vi "SaveStep.vi"(11 "Cluster":T2) -> (1 "StepForward":T1(ring), 2 "StepBack":T1(ring), 3 "Cluster":T2)   [LabVIEW 2021, in "Tree.lvlib" / "Tree.lvclass"]
uses:
  Tree.lvclass
  TreeController.ctl
  TreeData.ctl
panel:
  out "Del index":i32
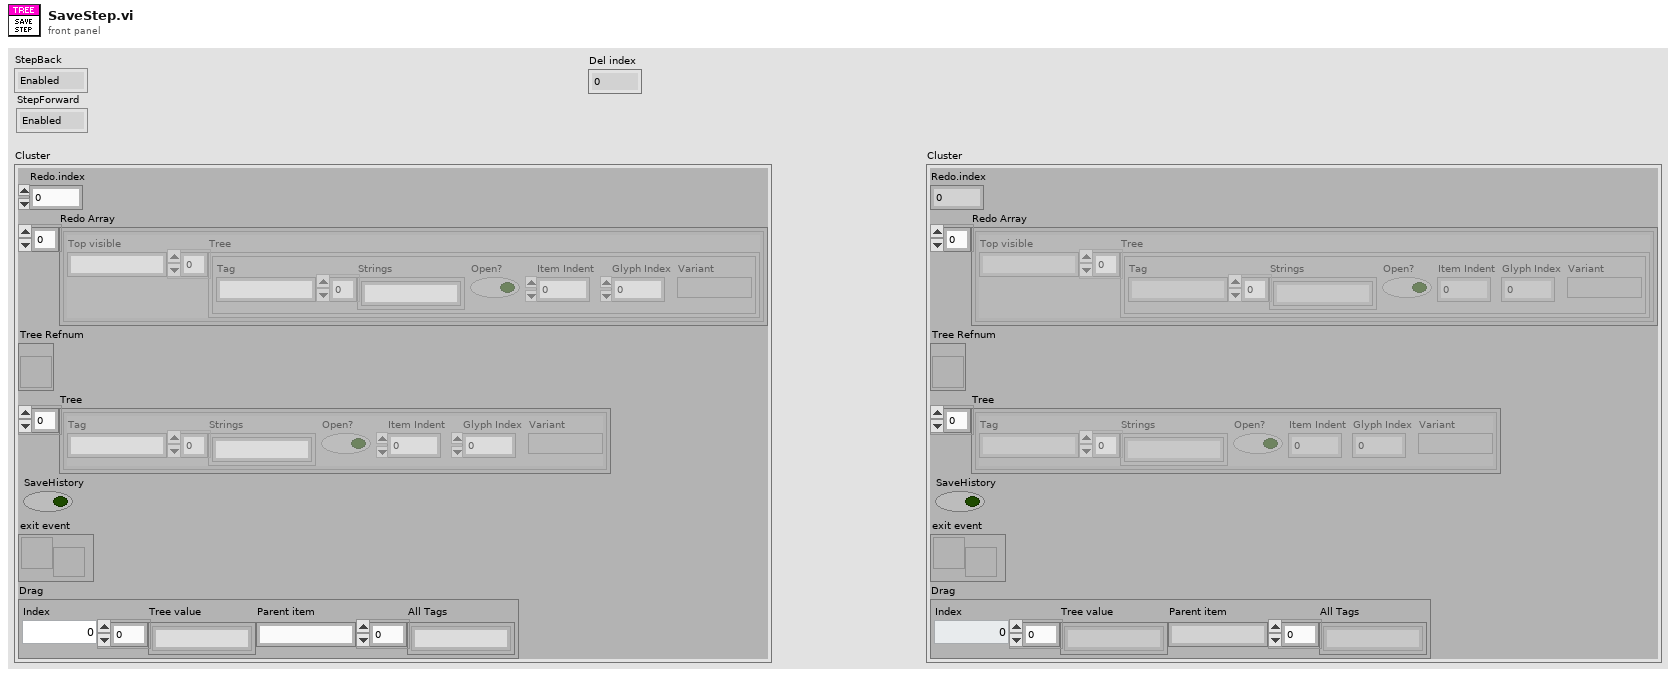
[diagram p1: front panel]
types:
  T1 = enum8{"Enabled", "Disabled", "Disabled and Grayed Out"}
  T2 = typedef "Tree.lvlib/Tree.lvclass/TreeController.ctl" = cluster{"Redo.index":i32, "Redo Array":cluster{"Top visible":string, "Tree":T3[]}[], "Tree Refnum":refnum<vi>, "Tree":T3[], "SaveHistory":bool, "exit event":refnum<user-event>, "Drag":cluster{"Index":i32, "Tree value":string[], "Parent item":string, "All Tags":string[]}}
  T3 = typedef "Tree.lvlib/Tree.lvclass/TreeData.ctl" = cluster{"Tag":string, "Strings":string[], "Open?":bool, "Item Indent":i32, "Glyph Index":i32, "Variant":variant}
  T4 = typedef "LVNodeAndColumnTypeDef.ctl" = cluster{"Node":string, "Column":i32}
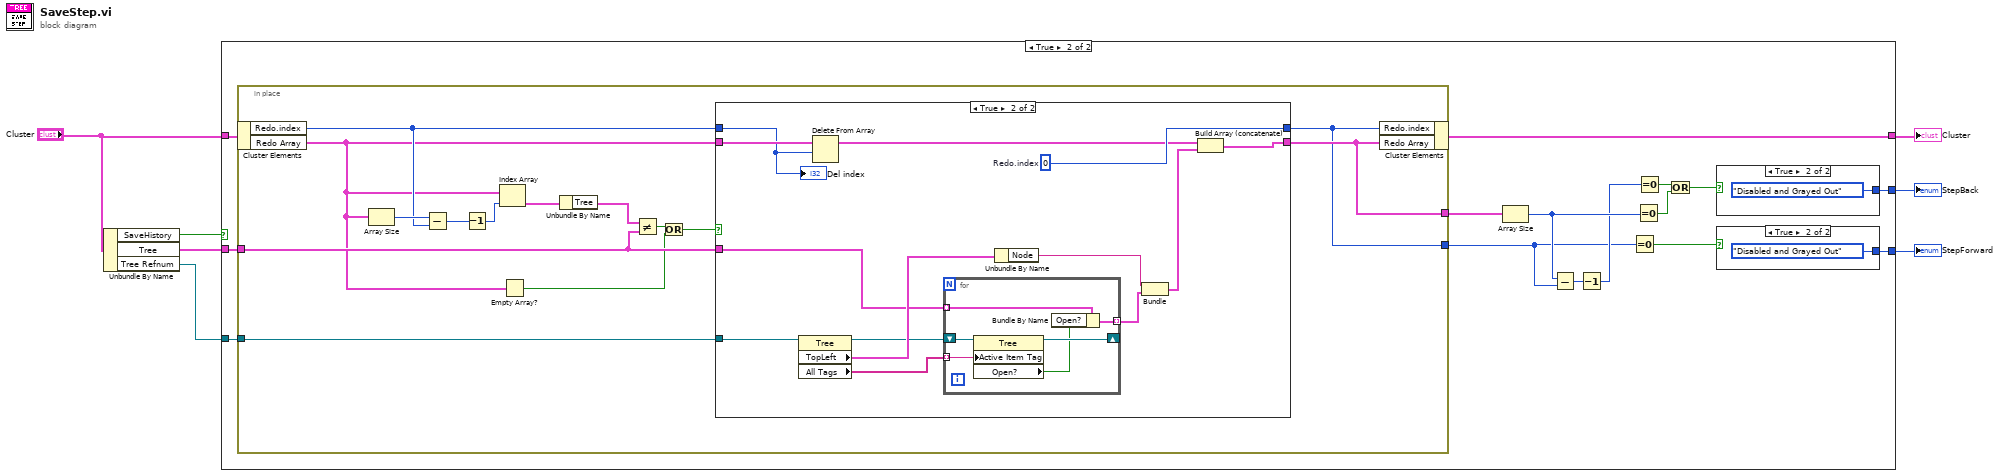
[diagram p0: block diagram]
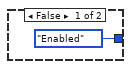
[diagram p3: hidden frame]
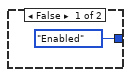
[diagram p4: hidden frame]
diagram:
  n1 = Unbundle By Name("Cluster") -> ("SaveHistory"=w2:bool, "Tree"=w7:T3[], "Tree Refnum"=w1:refnum<vi>)
  n2 = case shown="True" w2 {
    tunnel: w7 -> [_ w23]
    tunnel: "Cluster" -> [w8 w22]
    tunnel: [w8 w21] -> w5
    tunnel: w1 -> [_ w20]
    tunnel: [_ w10] -> w4
    tunnel: [_ w9] -> w3
    frame False {
    }
    frame True {
      n3 = in-place {
        in-place-border: w23 -> [w35]
        in-place-border: w20 -> [w38]
        in-place-border: [w33] -> w12
        in-place-border: [w32] -> w11
        n4 = in-place-cluster #1(w22) -> ("Redo.index"=w34:i32, "Redo Array"=w31:cluster{"Top visible":string, "Tree":T3[]}[])
        n5 = Array Size(array=w31) -> (size(s)=w39:i32)
        n6 = Subtract(x=w39, y=w34) -> (x-y=w40:i32)
        n7 = Decrement(x=w40) -> (x-1=w41:i32)
        n8 = Index Array(array=w31, index=w41) -> (element=w37:cluster{"Top visible":string, "Tree":T3[]})
        n9 = Empty Array?(array=w31) -> (empty?=w30:bool)
        n10 = Unbundle By Name(w37) -> ("Tree"=w36:T3[])
        n11 = Not Equal?(x=w36, y=w35) -> (x != y?=w29:bool)
        n12 = Or(x=w29, y=w30) -> (x .or. y?=w28:bool)
        n13 = case shown="True" w28 {
          tunnel: [w43 w56] -> w32
          tunnel: w31 -> [w42 w48]
          tunnel: w38 -> [_ w51]
          tunnel: [w42 w49] -> w33
          tunnel: w35 -> [_ w45]
          tunnel: w34 -> [w43 w46]
          frame False {
          }
          frame True {
            w56 = 0  # Redo.index
            n14 = property class="Tree"(reference=w51) -> (reference out=w52:refnum<vi>, "TopLeft"=w55:T4, "All Tags"=w53:string[])  [unwired: 1 in, 1 out]
            n15 = Delete From Array(array=w48, length=w46) -> (array with subset deleted=w47:cluster{"Top visible":string, "Tree":T3[]}[])  [unwired: 1 in, 1 out]
            n16 = for {
              tunnel: w53 -> [w62] mode=indexing
              shift-right: [w60] -> _
              shift-left: w52 -> [w61]
              tunnel: w45 -> [w59] mode=indexing
              tunnel: [w57] -> w44 mode=indexing
              n17 = property class="Tree"(reference=w61, "Active Item Tag"=w62) -> (reference out=w60:refnum<vi>, "Open?"=w58:bool)  [unwired: 1 in, 1 out]
              n18 = Bundle By Name(cluster=w59, "Open?"=w58) -> (w57:T3)
            }
            n19 = Unbundle By Name(w55) -> ("Node"=w54:string)
            n20 = Bundle("Node"=w54, w44) -> (w50:cluster{"Node":string, T3[]})  [unwired: 1 in]
            n21 = Build Array (concatenate)(w47, w50) -> (w49:cluster{"Node":string, "Tree":T3[]}[])
            "Del index" <- w46
          }
        }
        n22 = in-place-cluster #1("Redo.index"=w32, "Redo Array"=w33) -> (w21:T2)
      }
      n23 = Array Size(array=w12) -> (size(s)=w16:i32)
      n24 = Subtract(x=w16, y=w11) -> (x-y=w15:i32)
      n25 = Decrement(x=w15) -> (x-1=w14:i32)
      n26 = Equal To 0?(x=w11) -> (x = 0?=w19:bool)
      n27 = Equal To 0?(x=w16) -> (x = 0?=w17:bool)
      n28 = Equal To 0?(x=w14) -> (x = 0?=w13:bool)
      n29 = Or(x=w13, y=w17) -> (x .or. y?=w18:bool)
      n30 = case shown="True" w18 {
        tunnel: [T1."Enabled" ("Disabled & Grayed") T1."Disabled and Grayed Out" ("Disabled & Grayed")] -> w10
        frame False {
        }
        frame True {
        }
      }
      n31 = case shown="True" w19 {
        tunnel: [T1."Enabled" ("Disabled & Grayed") T1."Disabled and Grayed Out" ("Disabled & Grayed")] -> w9
        frame False {
        }
        frame True {
        }
      }
    }
  }
  "Cluster" <- w5
  "StepBack" <- w4
  "StepForward" <- w3
